vi "test_alignRightValidationIgnoringLabels.vi"(11 "Test Case In":refnum<class "AlignmentTests.lvclass">) -> (0 "error out":errorcluster, 3 "Test Case Out":refnum<class "AlignmentTests.lvclass">)   [LabVIEW 2023, in "AlignmentTests.lvclass"]
uses:
  AlignmentTests.lvclass
  <vilib>/Astemes/LUnit/Test Case.lvclass/Test Case.ctl
  <vilib>/Astemes/LUnit/Core/LUnit Test Case/Private/Append Fail Result.vi
  <vilib>/Astemes/LUnit/Core/LUnit Test Case/Private/Append Pass Result.vi
  <vilib>/Astemes/LUnit/Core/LUnit Test Case/Private/Run In UI.vi
  <vilib>/Utility/error.llb/Clear Errors.vi
  AlignmentTests.lvclass/AlignmentTests.ctl
  <vilib>/Astemes/LUnit/Test Case.lvclass
panel:
  in  "Numeric 3":dbl
  in  "Numeric 2_long catption":dbl
  in  "Numeric 1 long caption":dbl caption="Numeric sdsad"
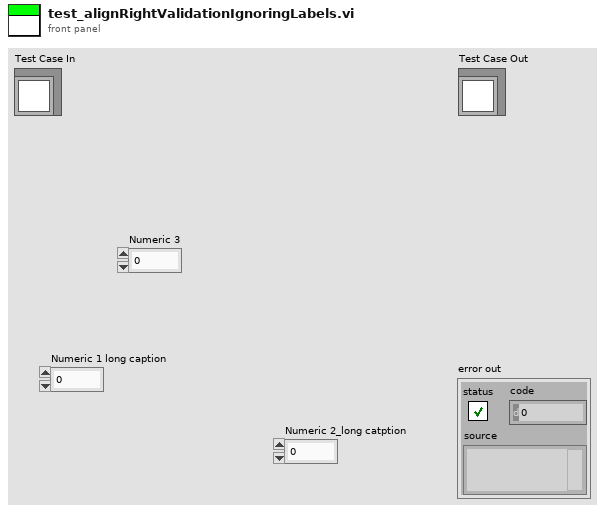
[diagram p1: front panel]
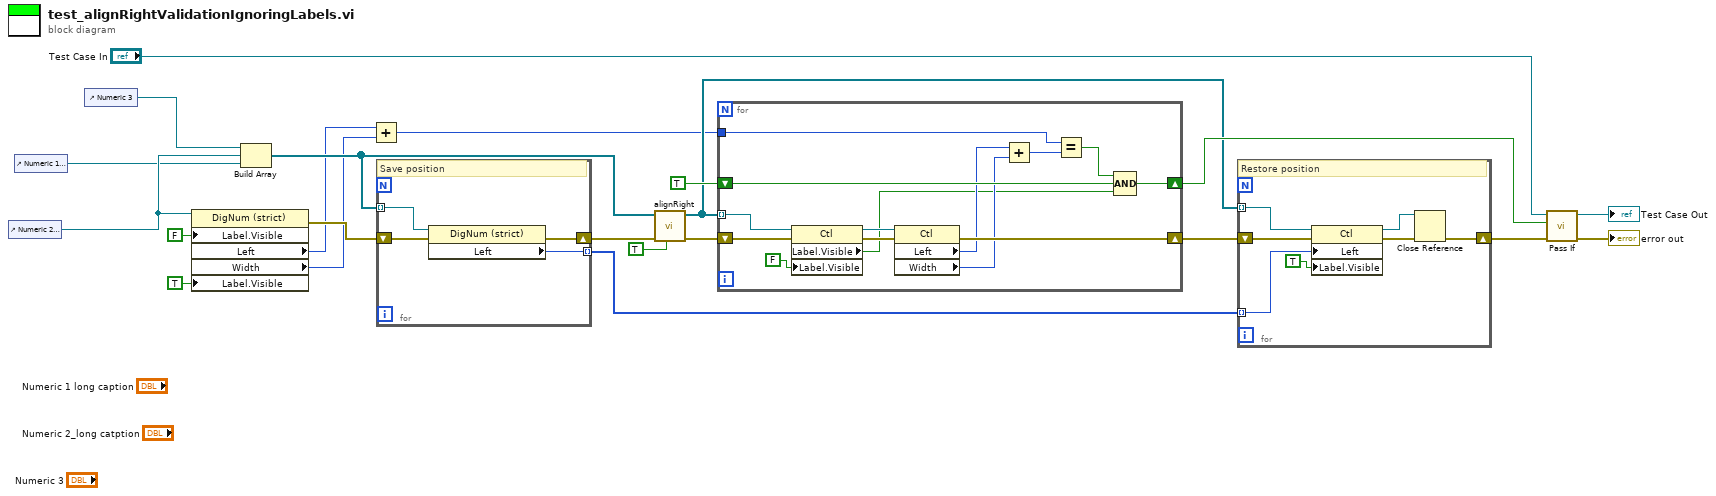
[diagram p0: block diagram]
diagram:
  n1 = control-ref of="Numeric 2_long catption"() -> (w18:refnum<vi>)
  n2 = control-ref of="Numeric 1 long caption"() -> (w17:refnum<vi>)
  n3 = control-ref of="Numeric 3"() -> (w19:refnum<vi>)
  n4 = property class="DigNum (strict)"(reference=w18, "Label.Visible"=FALSE, "Label.Visible"=TRUE) -> (error out=w13:errorcluster, "Left"=w5:i32, "Width"=w6:u32)  [unwired: 1 in, 1 out]
  n5 = Build Array(w19, w18, w17) -> (w8:refnum<vi>[])
  n6 = Add(x=w5, y=w6) -> (x+y=w4:u32)
  n7 = for {
    tunnel: w8 -> [w26] mode=indexing
    shift-right: [w24] -> w12
    shift-left: w13 -> [w25]
    tunnel: [w23] -> w9 mode=indexing
    # "Save position"
    n8 = property class="DigNum (strict)"(reference=w26, error in=w25) -> (error out=w24:errorcluster, "Left"=w23:i32)  [unwired: 1 out]
  }
  n9 = call "alignRight.vi"("useControlBodyOnly"=TRUE ("ignoreCaption&Labels"), "error in (no error)"=w12, "refs"=w8) -> ("error out"=w14:errorcluster, "refs(dup)"=w7:refnum<vi>[])  [unwired: 7 in]
  n10 = for {
    tunnel: w7 -> [w29] mode=indexing
    tunnel: w4 -> [w40]
    shift-right: [w38] -> w15
    shift-left: TRUE -> [w37]
    shift-right: [w36] -> w10
    shift-left: w14 -> [w32]
    n11 = property class="Ctl"(reference=w29, error in=w32, "Label.Visible"=FALSE) -> (reference out=w30:refnum<vi>, error out=w31:errorcluster, "Label.Visible"=w28:bool)
    n12 = property class="Ctl"(reference=w30, error in=w31) -> (error out=w36:errorcluster, "Left"=w34:i32, "Width"=w35:u32)  [unwired: 1 out]
    n13 = Add(x=w34, y=w35) -> (x+y=w33:u32)
    n14 = Equal?(x=w40, y=w33) -> (x = y?=w39:bool)
    n15 = Compound Arithmetic op=AND(w39, w37, w28) -> (w38:bool)
  }
  n16 = for {
    tunnel: w7 -> [w47] mode=indexing
    shift-right: [w43] -> w11
    shift-left: w10 -> [w46]
    tunnel: w9 -> [w44] mode=indexing
    # "Restore position"
    n17 = property class="Ctl"(reference=w47, error in=w46, "Left"=w44, "Label.Visible"=TRUE) -> (reference out=w42:refnum<vi>, error out=w45:errorcluster)
    n18 = Close Reference(reference=w42, error in (no error)=w45) -> (error out=w43:errorcluster)
  }
  n19 = call <vilib>:"Pass If.vi"("error in (no error)"=w11, "Pass?"=w15, "LUnit Test Case In"="Test Case In") -> ("error out"=→"error out":errorcluster, "LUnit Test Case Out"=→"Test Case Out":refnum<class "AlignmentTests.lvclass">)  [unwired: 7 in]
